vi "Publish Setpoint.vi"(8 "error in":errorcluster, 10 "Ident":string, 11 "Task Actor in":refnum<class "Task Actor.lvclass">) -> (0 "error out":errorcluster, 3 "Task Actor out":refnum<class "Task Actor.lvclass">)   [LabVIEW 2024, in "Task Actor.lvlib" / "Task Actor.lvclass"]
uses:
  Task Actor.lvclass
  <vilib>/ActorFramework/Actor/Actor.lvclass/Actor.ctl
  Task Actor.lvclass/Task Actor.ctl
  Series/ISeries Actor/ISeries Actor Messages/Task Setpoint Updated Msg/Task Setpoint Updated Msg.lvclass/Task Setpoint Updated Msg.ctl
  <vilib>/ActorFramework/Message Enqueuer/Message Enqueuer.lvclass/Message Enqueuer.ctl
  <vilib>/ActorFramework/Message Enqueuer/Enqueue.vi
  Series/ISeries Actor/ISeries Actor Messages/Task Setpoint Updated Msg/Task Setpoint Updated Msg.lvclass
  <vilib>/Utility/LVClass/Get LV Class Name.vi
  <resource>/AFDebug/Generate Trace for Message.vi
  <vilib>/ActorFramework/Message Priority Queue/Priority Enqueue.vi
  <vilib>/ActorFramework/Actor/Actor.lvclass
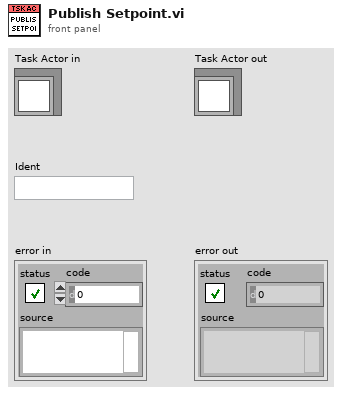
[diagram p1: front panel]
types:
  T1 = map{string, cluster{"New?":bool, "Data":variant}}
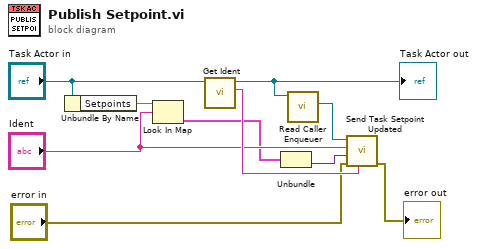
[diagram p0: block diagram]
diagram:
  n1 = Unbundle By Name("Task Actor in") -> ("Setpoints"=w10:T1)
  n2 = Look In Map(map=w10, key="Ident") -> (value=w4:cluster{"Processed?":bool, "Data":variant})  [unwired: 1 in, 1 out]
  n3 = call "Get Ident.vi"("Task Actor in"="Task Actor in") -> ("Ident"=w6:string, "Task Actor out"=w7:refnum<class "Task Actor.lvclass">)  [unwired: 9 in]
  "Task Actor out" <- w7
  n4 = Unbundle(w4) -> ("Data"=w1:variant)  [unwired: 1 out]
  n5 = call <vilib>:"Read Caller Enqueuer.vi"("Actor"=w7) -> ("Caller Enqueuer"=w8:refnum<class "Message Enqueuer.lvclass">)  [unwired: 10 in]
  n6 = call "Send Task Setpoint Updated.vi"("Task Ident"=w6, "error in (no error)"="error in", "Data"=w1, "Setpoint Ident"="Ident", "Message Enqueuer"=w8) -> ("error out"=→"error out":errorcluster)  [unwired: 5 in, 1 out]
